vi "SP Select Current Plot.vi"(1 "Plots Tab Control":refnum<vi>, 3 "Selected? Ref":refnum<vi>) -> (0 "Plot Ref":refnum<vi>)   [LabVIEW 2011]
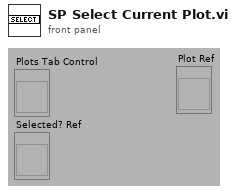
[diagram p1: front panel]
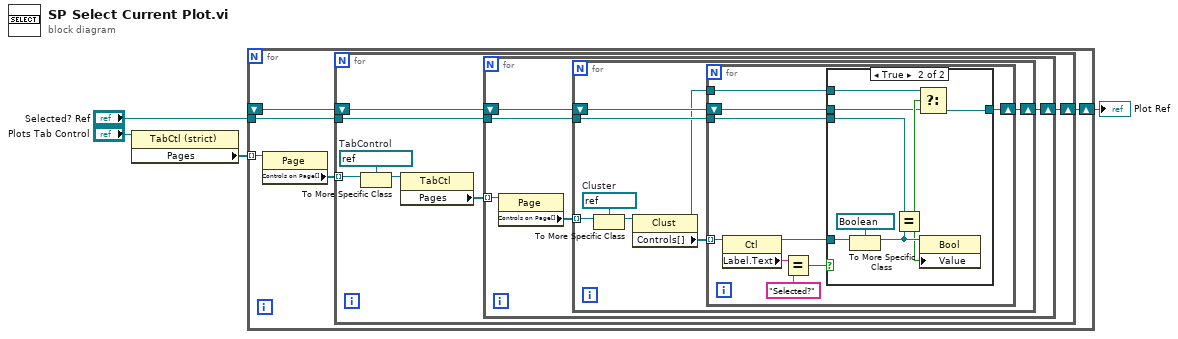
[diagram p0: block diagram]
diagram:
  n1 = property class="TabCtl (strict)"(reference="Plots Tab Control") -> ("Pages"=w2:refnum<vi>[])  [unwired: 1 in, 2 out]
  n2 = for {
    tunnel: w2 -> [w6] mode=indexing
    tunnel: "Selected? Ref" -> [w9]
    shift-right: [w7] -> w3
    shift-left: _ -> [w8]
    n3 = property class="Page"(reference=w6) -> ("Controls on Page[]"=w5:refnum<vi>[])  [unwired: 1 in, 2 out]
    n4 = for {
      tunnel: w9 -> [w16]
      tunnel: w5 -> [w13] mode=indexing
      shift-right: [w14] -> w7
      shift-left: w8 -> [w15]
      w12 = refnum<vi> refnum  # TabControl
      n5 = To More Specific Class(target class=w12, reference=w13) -> (specific class reference=w11:refnum<vi>)  [unwired: 1 in, 1 out]
      n6 = property class="TabCtl"(reference=w11) -> ("Pages"=w10:refnum<vi>[])  [unwired: 1 in, 2 out]
      n7 = for {
        tunnel: w16 -> [w21]
        tunnel: w10 -> [w18] mode=indexing
        shift-right: [w19] -> w14
        shift-left: w15 -> [w20]
        n8 = property class="Page"(reference=w18) -> ("Controls on Page[]"=w17:refnum<vi>[])  [unwired: 1 in, 2 out]
        n9 = for {
          tunnel: w21 -> [w29]
          tunnel: w17 -> [w25] mode=indexing
          shift-right: [w27] -> w19
          shift-left: w20 -> [w28]
          w26 = refnum<vi> refnum  # Cluster
          n10 = To More Specific Class(target class=w26, reference=w25) -> (specific class reference=w24:refnum<vi>)  [unwired: 1 in, 1 out]
          n11 = property class="Clust"(reference=w24) -> (reference out=w22:refnum<vi>, "Controls[]"=w23:refnum<vi>[])  [unwired: 1 in, 1 out]
          n12 = for {
            tunnel: w23 -> [w36] mode=indexing
            tunnel: w29 -> [w33]
            tunnel: w22 -> [w32]
            shift-right: [w30] -> w27
            shift-left: w28 -> [w31]
            n13 = property class="Ctl"(reference=w36) -> (reference out=w34:refnum<vi>, "Label.Text"=w38:string)  [unwired: 1 in, 1 out]
            n14 = Equal?(x=w38, y="Selected?") -> (x = y?=w35:bool)
            n15 = case shown="True" w35 {
              tunnel: w34 -> [_ w45]
              tunnel: w33 -> [_ w47]
              tunnel: w32 -> [_ w42]
              tunnel: w31 -> [w39 w41]
              tunnel: [w39 w40] -> w30
              frame False {
              }
              frame True {
                n16 = To More Specific Class(target class=refnum<vi> refnum ("Selected? Ref"), reference=w45) -> (specific class reference=w44:refnum<vi>)  [unwired: 1 in, 1 out]
                n17 = Equal?(x=w47, y=w44) -> (x = y?=w43:bool)
                n18 = Select(t=w42, s=w43, f=w41) -> (s? t:f=w40:refnum<vi>)
                n19 = property class="Bool"(reference=w44, "Value"=w43) -> ()  [unwired: 1 in, 2 out]
              }
            }
          }
        }
      }
    }
  }
  "Plot Ref" <- w3
